vi "PicoReleaseMultiBuffers.vi"(8 "error in (no error)":errorcluster, 9 "Enabled array":i16[](array[numeric]), 10 "Data Pointers":T1) -> (0 "error out":errorcluster, 2 "Data Pointers Out":T1)   [LabVIEW 2024]
doc: "Release Picodata buffers for Block and 6000a streaming examples"
uses:
  PicoBuffers.ctl
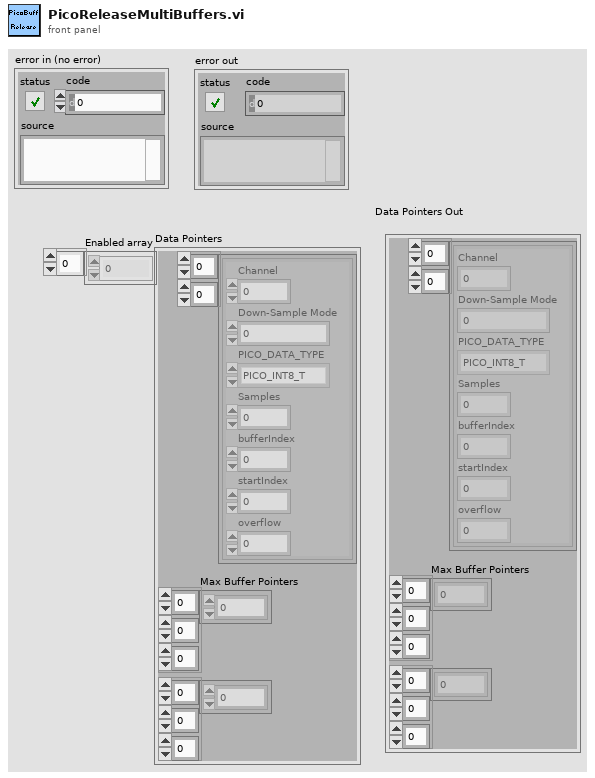
[diagram p1: front panel]
types:
  T1 = typedef "PicoBuffers.ctl" = cluster{"Max Buffer Pointers":u64[][][], "Min Buffer Pointers":u64[][][], "StreamingDataInfo":cluster{"Channel":u32, "Down-Sample Mode":u32, "PICO_DATA_TYPE":enum32{"PICO_INT8_T", "PICO_INT16_T", "PICO_INT32_T", "PICO_UINT32_T", "PICO_INT64_T", ""}, "Samples":i32, "bufferIndex":u64, "startIndex":i32, "overflow":i16}[][]}
  T2 = cluster{"status":bool, "code":bool, "source":bool}
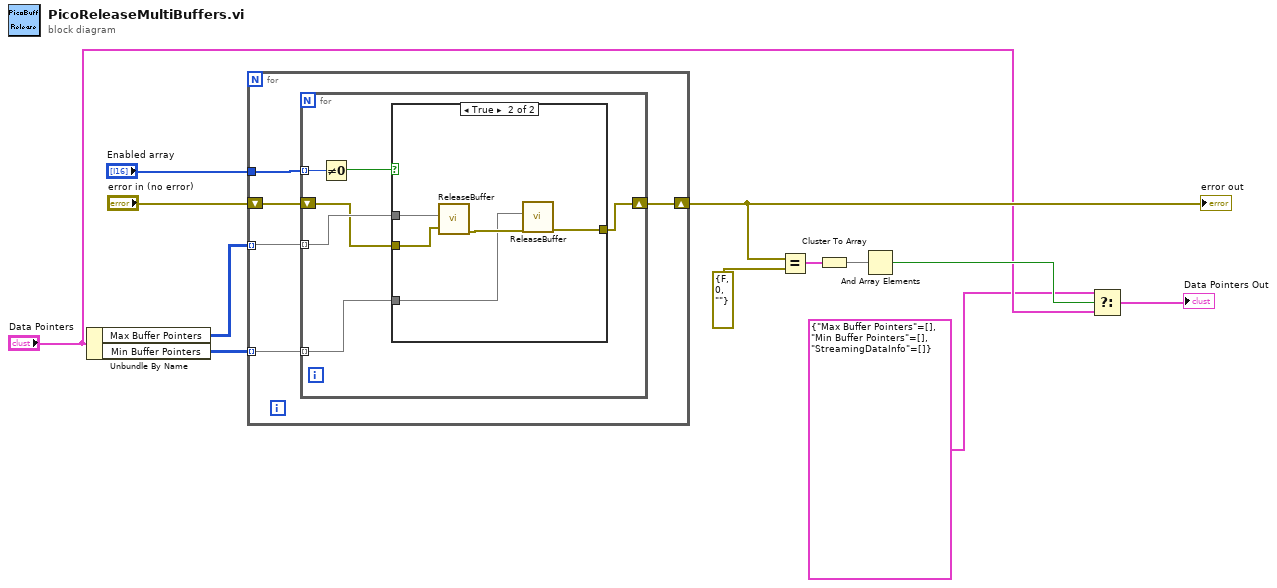
[diagram p0: block diagram]
diagram:
  n1 = Unbundle By Name("Data Pointers") -> ("Max Buffer Pointers"=w10:u64[][][], "Min Buffer Pointers"=w9:u64[][][])
  n2 = for {
    tunnel: w10 -> [w17] mode=indexing
    shift-right: [w15] -> w7
    shift-left: "error in (no error)" -> [w16]
    tunnel: "Enabled array" -> [w14]
    tunnel: w9 -> [w13] mode=indexing
    n3 = for {
      tunnel: w17 -> [w23] mode=indexing
      tunnel: w14 -> [w22] mode=indexing
      shift-right: [w20] -> w15
      shift-left: w16 -> [w21]
      tunnel: w13 -> [w19] mode=indexing
      n4 = Not Equal To 0?(x=w22) -> (x != 0?=w18:bool)
      n5 = case shown="True" w18 {
        tunnel: w23 -> [_ w29]
        tunnel: w21 -> [w24 w28]
        tunnel: [w24 w26] -> w20
        tunnel: w19 -> [_ w25]
        frame False {
        }
        frame True {
          n6 = call "ReleaseBuffer.vi"("error in (no error)"=w28, "Pointer and BufferSize"=w29) -> ("error out"=w27:errorcluster)  [unwired: 9 in]
          n7 = call "ReleaseBuffer.vi"("error in (no error)"=w27, "Pointer and BufferSize"=w25) -> ("error out"=w26:errorcluster)  [unwired: 9 in]
        }
      }
    }
  }
  "error out" <- w7
  n8 = Equal?(x=w7, y=errorcluster {"status"=FALSE, "code"=0, "source"=""} ("error constant")) -> (x = y?=w5:T2)
  n9 = Cluster To Array(cluster=w5) -> (array=w4:bool[])
  n10 = And Array Elements(Boolean array=w4) -> (logical AND=w3:bool)
  n11 = Select(t=T1 {"Max Buffer Pointers"=[], "Min Buffer Pointers"=[], "StreamingDataInfo"=[]} ("Data Pointers"), s=w3, f="Data Pointers") -> (s? t:f=→"Data Pointers Out":T1)
